vi "MilanTest.vi"() -> ()   [LabVIEW 2020]
uses:
  Subs/Server XCtrl/Server.xctl
  Subs/ColorText/Code.xctl
  Subs/SystemLink/SL_Subs/SL_XControl.xctl
panel:
  in  "SL_XControl":string(xcontrol)
  in  "Code":string(xcontrol)="import hub,utime\nfred = hub.USB_VCP()\n\nrequest = b'urequest(\"apple.com\")'\neol = b'web'\nreol = b'back'\n\ndef comm(b_string):\n    s =  b''\n    fred.write(b_string + eol)\n    while not(reol in s):\n        try:\n            s = s + fred.readline()\n        except:\n            utime.sleep(0.1)\n    # print(s)\n\ncomm(request)\n\ns =  b''\nfred.write(b_string + eol)\n    while not(reol in s):\n        try:\n            s = s + fred.readline()\n        except:\n            utime.sleep(0.1)\n       print(s)\n    \n"
  in  "Server":path(xcontrol)=path "/Users/crogers/GitHub/Summer2020/LabVIEWCode/Servers/Jens.vi"
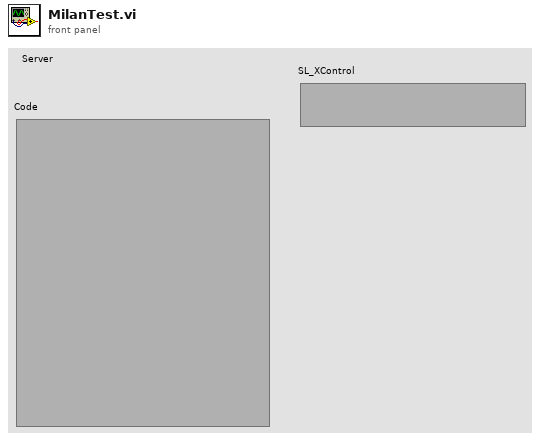
[diagram p1: front panel]
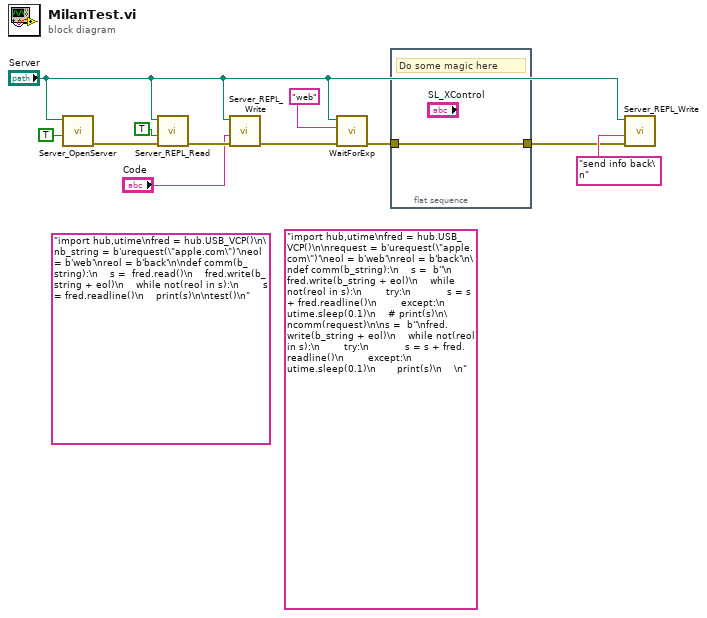
[diagram p0: block diagram]
diagram:
  (unwired) "import hub,utime\nfred = hub.USB_VCP()\n\nrequest = b'urequest(\"apple.com\")'\neol = b'web'\nreol = b'back'\n\ndef comm(b_string):\n    s =  b''\n    fred.write(b_string + eol)\n    while not(reol in s):\n        try:\n            s = s + fred.readline()\n        except:\n            utime.sleep(0.1)\n    # print(s)\n\ncomm(request)\n\ns =  b''\nfred.write(b_string + eol)\n    while not(reol in s):\n        try:\n            s = s + fred.readline()\n        except:\n            utime.sleep(0.1)\n       print(s)\n    \n" ("Code")
  (unwired) "import hub,utime\nfred = hub.USB_VCP()\n\nb_string = b'urequest(\"apple.com\")'\neol = b'web'\nreol = b'back'\n\ndef comm(b_string):\n    s =  fred.read()\n    fred.write(b_string + eol)\n    while not(reol in s):\n        s = fred.readline()\n    print(s)\n\ntest()\n" ("Code")
  n1 = call "Server_OpenServer.vi"("Wait for connection?"=TRUE, "Server"="Server") -> ("error out"=w9:errorcluster)  [unwired: 9 in]
  n2 = call "Server_REPL_Read.vi"("error in (no error)"=w9, "Clear"=TRUE, "Server"="Server") -> ("error out"=w8:errorcluster)  [unwired: 6 in, 2 out]
  n3 = call "Server_REPL_Write.vi"("error in (no error)"=w8, "Code"="Code", "Server"="Server") -> ("error out"=w11:errorcluster)  [unwired: 8 in]
  n4 = call "WaitForExp.vi"("error in (no error)"=w11, "expression"="web" ("regular expression"), "Server"="Server") -> ("error out"=w2:errorcluster)  [unwired: 7 in, 1 out]
  n5 = flat-sequence {
    tunnel: [w12] -> w3
    tunnel: w2 -> [w12]
    frame #0 {
      # "Do some magic here"
    }
  }
  n6 = call "Server_REPL_Write.vi"("error in (no error)"=w3, "Code"="send info back\n" ("Command"), "Server"="Server") -> ()  [unwired: 8 in, 1 out]
